vi "Check Proxy Dll Existance.vi"(8 "error in (no error)":errorcluster, 11 "Proxy Dll Path":path) -> (0 "error out":errorcluster, 1 "Existing?":bool, 2 "Overwrite?":bool=TRUE, 3 "Proxy Dll Path (out)":path)   [LabVIEW 2020, in "WebServiceImporter.lvlib" / "Main Panel.lvlib" / "Input Info.lvlib"]
doc: "Check whether the local proxy dll indicated by \"Proxy Dll Path\" exists. \"Overwrite\" will be set to FALSE only when:\n1) The indicated local proxy dll already exists.\n2) The user choose not to overwrite the exist one in the prompt dialog."
uses:
  <vilib>/Platform/WebService/Main Panel/Pages/Input Info/Input Info.lvlib
  <vilib>/Platform/WebService/Global/Const Strings.vi
  <vilib>/Platform/WebService/WebServiceImporter.lvlib
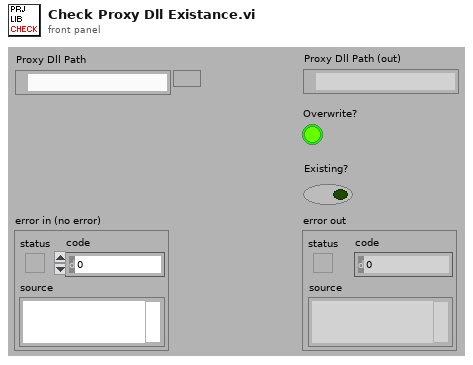
[diagram p1: front panel]
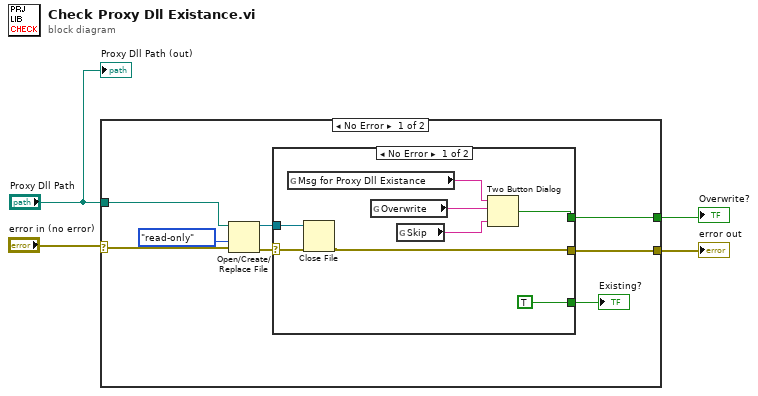
[diagram p0: block diagram]
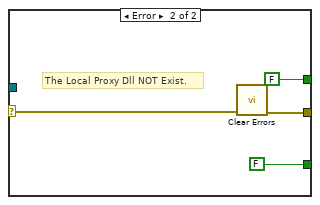
[diagram p2: hidden frame]
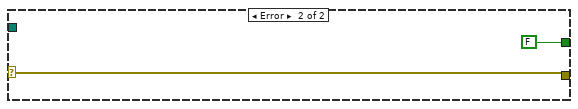
[diagram p3: hidden frame]
diagram:
  n1 = case shown="No Error" "error in (no error)" {
    selector: "error in (no error)" -> [w12 w26]
    tunnel: "Proxy Dll Path" -> [w10 _]
    tunnel: [w7 w26] -> w2
    tunnel: [w6 FALSE] -> w1
    frame No Error {
      n2 = Open/Create/Replace File(file path (use dialog)=w10, error in=w12, access (0:read/write)=enum16{"read/write", "read-only", "write-only"}."read-only") -> (refnum out=w8:refnum<file>, error out=w9:errorcluster)  [unwired: 3 in, 1 out]
      n3 = case shown="No Error" w9 {
        selector: w9 -> [w19 w24]
        tunnel: w8 -> [w18 _]
        tunnel: [w17 w23] -> w7
        tunnel: [w20 FALSE] -> w6
        tunnel: [TRUE FALSE] -> w5
        frame No Error {
          n4 = global read "Const Strings.vi" "Msg for Proxy Dll Existance"() -> (w16:string)
          n5 = Close File(refnum=w18, error in=w19) -> (error out=w17:errorcluster)  [unwired: 1 out]
          n6 = global read "Const Strings.vi" "Overwrite"() -> (w15:string)
          n7 = global read "Const Strings.vi" "Skip"() -> (w14:string)
          n8 = Two Button Dialog(message=w16, 1:w14, 2:w15) -> (T button?=w20:bool)
        }
        frame Error {
          # "The Local Proxy Dll NOT Exist."
          n9 = call <vilib>:"Clear Errors.vi"("error in (no error)"=w24) -> ("error out"=w23:errorcluster)  [unwired: 5 in, 1 out]
        }
      }
      "Existing?" <- w5
    }
    frame Error {
    }
  }
  "error out" <- w2
  "Overwrite?" <- w1
  "Proxy Dll Path (out)" <- "Proxy Dll Path"
